vi "Curtin1_AddTest.vi"(10 "Old Files":T1[](array[typedef]), 11 "Selected Paths":path[](array[path])) -> (3 "New Files":T1[](array[typedef]))   [LabVIEW 2022 SP3]
uses:
  Curtin1_Label.ctl
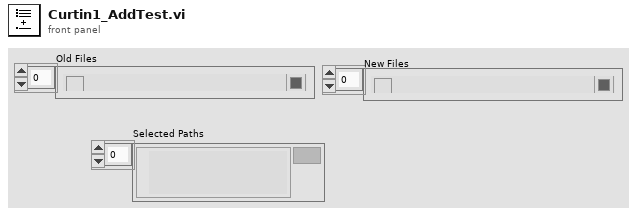
[diagram p1: front panel]
types:
  T1 = typedef "Curtin1_Label.ctl" = cluster{"Show?":bool, "Name":string, "Color":u32, "Path":path, "Show Notes":bool}
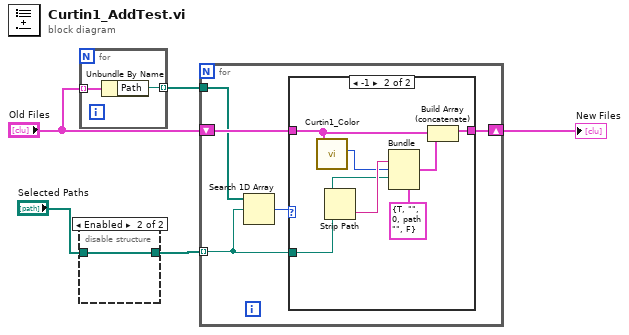
[diagram p0: block diagram]
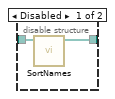
[diagram p2: hidden frame]
diagram:
  n1 = for {
    tunnel: "Old Files" -> [w7] mode=indexing
    tunnel: [w6] -> w4 mode=indexing
    n2 = Unbundle By Name(w7) -> ("Path"=w6:path)
  }
  n3 = disable-structure shown="Enabled" {
    disable-tunnel: "Selected Paths" -> [w9 w10]
    disable-tunnel: [w8 w10] -> w1
    frame Disabled {
      n4 = call "SortNames.vi"("Selected Paths"=w9) -> ("Selected Paths out"=w8:path[])  [unwired: 10 in]
    }
    frame Enabled {
    }
  }
  n5 = for {
    tunnel: w1 -> [w12] mode=indexing
    shift-right: [w15] -> w3
    shift-left: "Old Files" -> [w14]
    tunnel: w4 -> [w13]
    n6 = Search 1D Array(1D array=w13, element=w12) -> (index of element=w11:i32)  [unwired: 1 in]
    n7 = case shown="-1" w11 {
      tunnel: [w16 w23] -> w15
      tunnel: w14 -> [w16 w19]
      tunnel: w12 -> [_ w17]
      frame Default {
      }
      frame -1 {
        n8 = call "Curtin1_Color.vi"("Files in"=w19) -> ("New color"=w18:u32)  [unwired: 9 in, 1 out]
        n9 = Strip Path(path=w17) -> (name=w21:string)  [unwired: 1 out]
        n10 = Bundle(cluster=T1 {"Show?"=TRUE, "Name"="", "Color"=0, "Path"=path "", "Show Notes"=FALSE} ("Cluster"), "Name"=w21, "Color"=w18, "Path"=w17) -> (w22:T1)  [unwired: 2 in]
        n11 = Build Array (concatenate)(w19, w22) -> (w23:T1[])
      }
    }
  }
  "New Files" <- w3
